vi "Find CD Install Directory.vi"(8 "error in":errorcluster, 11 "consumer data":T1) -> (0 "error out":errorcluster, 1 "engine path":string, 2 "cd install directory":string, 3 "consumer data out":T1)   [LabVIEW 2020, in "Template Tool.lvlib"]
uses:
  Template Tool.lvlib
  Consumer Data.ctl
  Project Build Specs.ctl
  <vilib>/regexp/Match Regular Expression.xnode
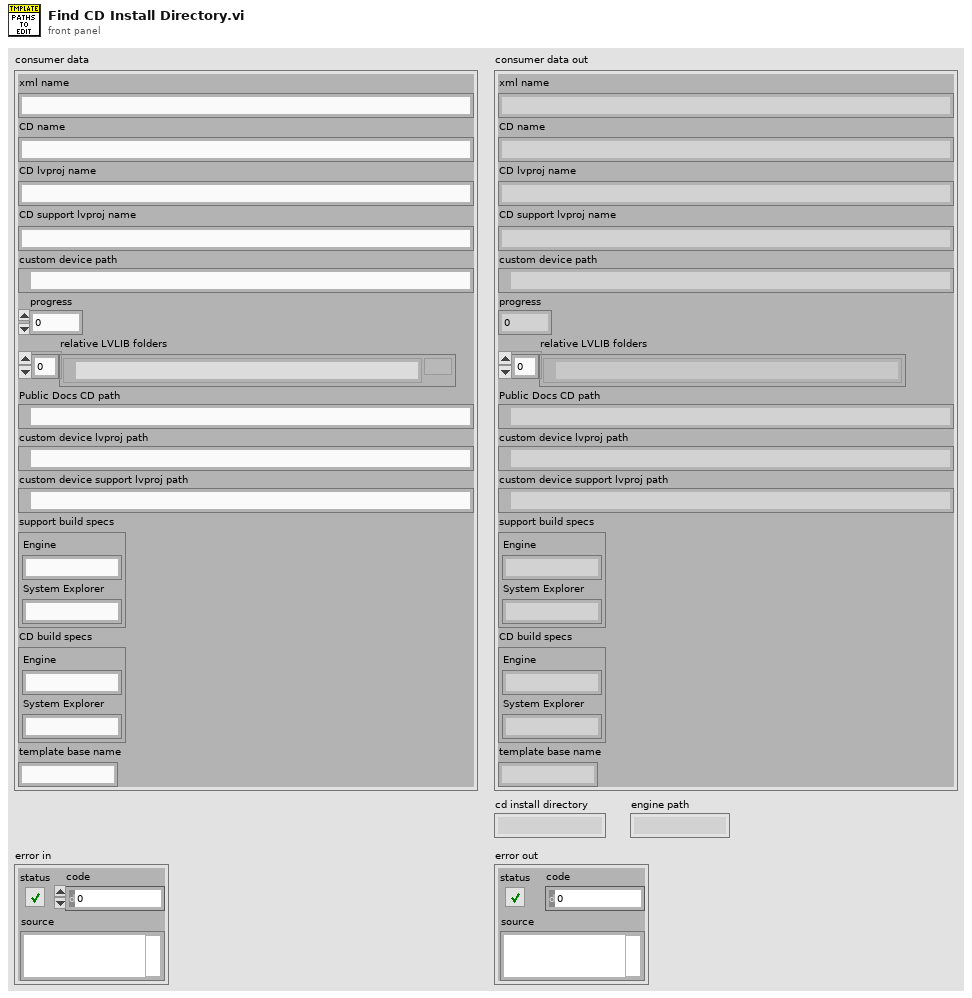
[diagram p1: front panel]
types:
  T1 = typedef "Template Tool.lvlib/Consumer Data.ctl" = cluster{"xml name":string, "CD name":string, "CD lvproj name":string, "CD support lvproj name":string, "custom device path":path, "progress":u8, "relative LVLIB folders":path[], "Public Docs CD path":path, "custom device lvproj path":path, "custom device support lvproj path":path, "support build specs":T2, "CD build specs":T2, "template base name":string}
  T2 = typedef "Template Tool.lvlib/Project Build Specs.ctl" = cluster{"Engine":string, "System Explorer":string}
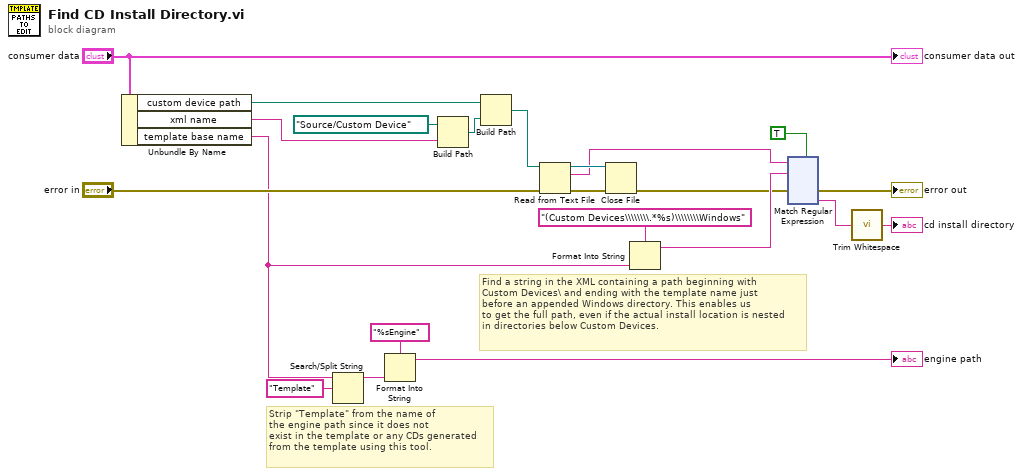
[diagram p0: block diagram]
diagram:
  # "Strip \"Template\" from the name of\nthe engine path since it does not\nexist in the template or any CDs generated\nfrom the template using this tool."
  # "Find a string in the XML containing a path beginning with\nCustom Devices\\ and ending with the template name just\nbefore an appended Windows directory. This enables us\nto get the full path, even if the actual install location is nested\nin directories below Custom Devices."
  n1 = Unbundle By Name("consumer data") -> ("custom device path"=w9:path, "xml name"=w7:string, "template base name"=w5:string)
  n2 = Search/Split String(string=w5, search string/char (-)="Template") -> (substring before match=w2:string)  [unwired: 1 in, 2 out]
  n3 = Format Into String(format string="%sEngine", w2) -> (resulting string=→"engine path":string)  [unwired: 2 in, 1 out]
  n4 = Build Path(base path=path "Source/Custom Device", name or relative path=w7) -> (appended path=w6:path)
  n5 = Build Path(base path=w9, name or relative path=w6) -> (appended path=w22:path)
  n6 = Read from Text File(file (use dialog)=w22, error in="error in") -> (refnum out=w19:refnum<file>, text=w15:string, error out=w20:errorcluster)  [unwired: 2 in, 1 out]
  n7 = Close File(refnum=w19, error in=w20) -> (error out=w12:errorcluster)  [unwired: 1 out]
  n8 = Format Into String(format string="(Custom Devices\\\\\\\\.*%s)\\\\\\\\Windows" ("search string"), w5) -> (resulting string=w16:string)  [unwired: 2 in, 1 out]
  n9 = xnode "Match Regular Expression"("input string"=w15, "regular expression"=w16, "error in"=w12, "multiline? (F)"=TRUE) -> ("error out"=→"error out":errorcluster, "submatch 1"=w14:string)  [unwired: 2 in, 4 out]
  n10 = call <vilib>:"Trim Whitespace.vi"("string"=w14) -> ("trimmed string"=→"cd install directory":string)  [unwired: 1 in]
  "consumer data out" <- "consumer data"
